vi "Fermeture VI.vi"   [LabVIEW 2020]
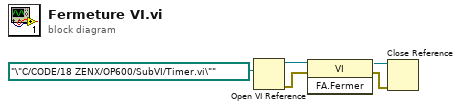
[diagram p0: block diagram]
diagram:
  n1 = Open VI Reference(vi path=path "/\"C/CODE/18 ZENX/OP600/SubVI/Timer.vi\"" ("chemin du VI")) -> (vi reference=w5:refnum<vi>, error out=w2:errorcluster)  [unwired: 5 in]
  n2 = invoke class="VI" method="FA.Fermer"(reference=w5, error in=w2) -> (reference out=w3:refnum<vi>, error out=w4:errorcluster)  [unwired: 1 in, 1 out]
  n3 = Close Reference(reference=w3, error in (no error)=w4) -> ()  [unwired: 1 out]
